vi "Wire Handle Messages Case.vi"(8 "error in (no error)":errorcluster, 11 "Getter Generator in":refnum<class "Getter Generator.lvclass">) -> (0 "error out":errorcluster, 3 "Getter Generator out":refnum<class "Getter Generator.lvclass">)   [LabVIEW 2020, in "Method Generation.lvlib" / "Getter Generator.lvclass"]
uses:
  Getter Generator.lvclass
  Getter Generator.lvclass/Getter Generator.ctl
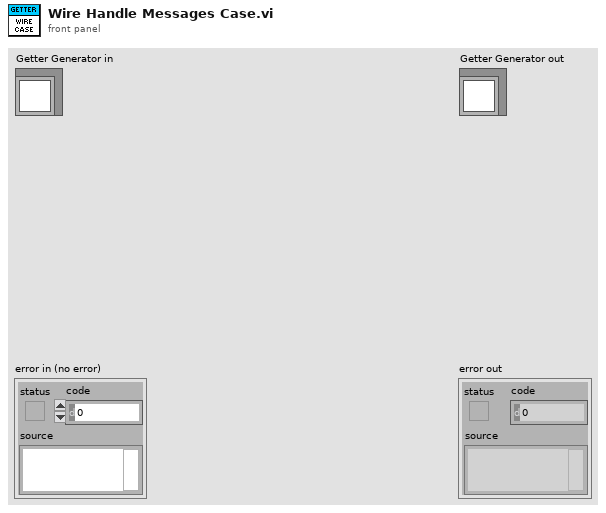
[diagram p1: front panel]
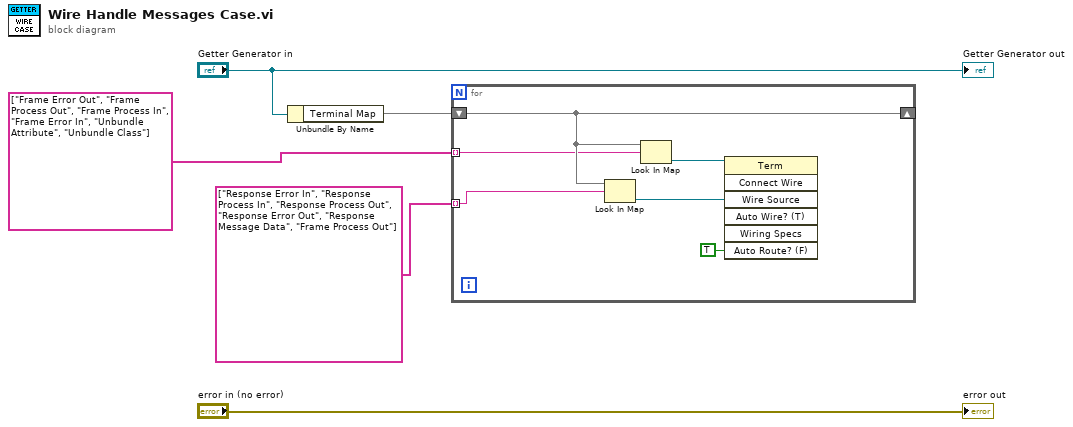
[diagram p0: block diagram]
diagram:
  n1 = Unbundle By Name("Getter Generator in") -> ("Terminal Map"=w3:map{string, refnum<vi>})
  n2 = for {
    shift-right: [w11] -> _
    shift-left: w3 -> [w11]
    tunnel: string[] ["Frame Error Out", "Frame Process Out", "Frame Process In", "Frame Error In", "Unbundle Attribute", "Unbundle Class"] ("key") -> [w10] mode=indexing
    tunnel: string[] ["Response Error In", "Response Process In", "Response Process Out", "Response Error Out", "Response Message Data", "Frame Process Out"] ("key") -> [w9] mode=indexing
    n3 = Look In Map(map=w11, key=w9) -> (value=w7:refnum<vi>)  [unwired: 1 in, 1 out]
    n4 = Look In Map(map=w11, key=w10) -> (value=w8:refnum<vi>)  [unwired: 1 in, 1 out]
    n5 = invoke class="Term" method="Connect Wire"(reference=w8, "Wire Source"=w7, "Auto Route? (F)"=TRUE) -> ()  [unwired: 4 in, 7 out]
  }
  "error out" <- "error in (no error)"
  "Getter Generator out" <- "Getter Generator in"
